vi "Default Settings.vi"(8 "error in (no error)":errorcluster, 11 "CAD Dispense2 in":refnum<class "CAD Dispense2.lvclass">) -> (0 "error out":errorcluster, 3 "CAD Dispense2 out":refnum<class "CAD Dispense2.lvclass">)   [LabVIEW 2016, in "CAD Dispense2.lvclass"]
uses:
  CAD Dispense2.lvclass
  D:/UCSB-Gantry_ms/UCSB-Gantry 0510/V5/Classes/Routine/Dispense/Dispense.lvclass
  CAD Dispense2.lvclass/CAD Dispense2.ctl
  Dispense.lvclass/Dispense.ctl
  Dispense.lvclass
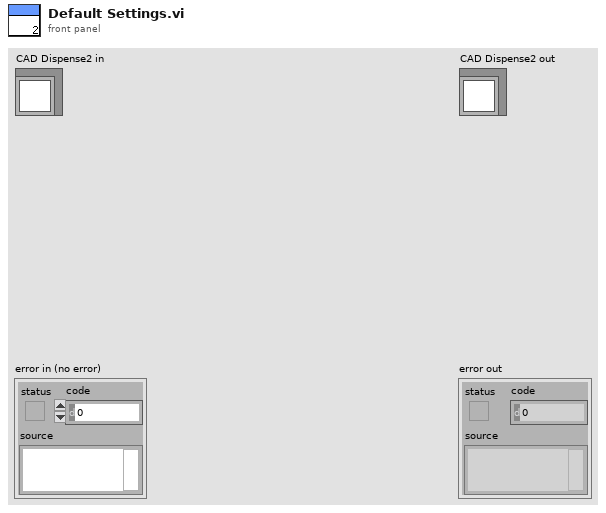
[diagram p1: front panel]
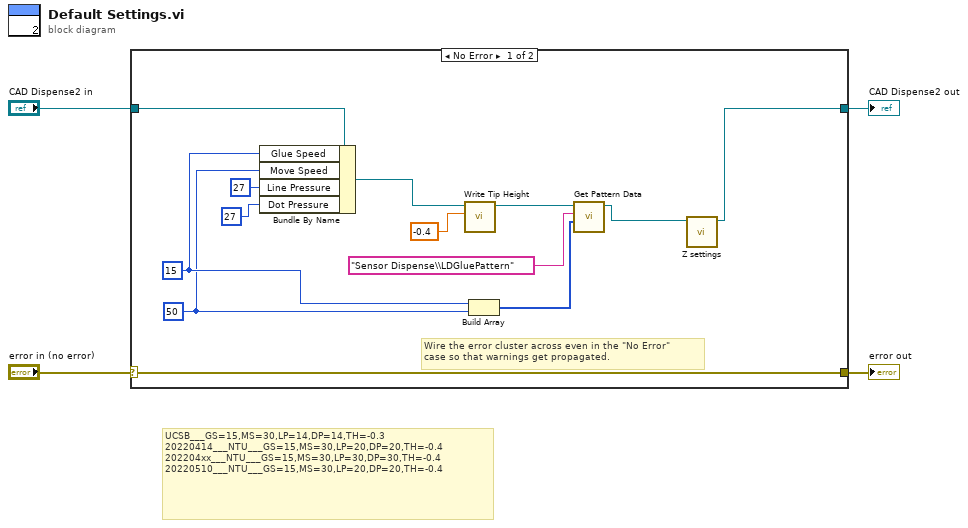
[diagram p0: block diagram]
diagram:
  # "UCSB___GS=15,MS=30,LP=14,DP=14,TH=-0.3\n20220414___NTU___GS=15,MS=30,LP=20,DP=20,TH=-0.4\n202204xx___NTU___GS=15,MS=30,LP=30,DP=30,TH=-0.4\n20220510___NTU___GS=15,MS=30,LP=20,DP=20,TH=-0.4"
  n1 = case shown="No Error" "error in (no error)" {
    selector: "error in (no error)" -> [w17 w19]
    tunnel: [w17 w19] -> w3
    tunnel: [w8 w18] -> w1
    tunnel: "CAD Dispense2 in" -> [w9 w18]
    frame No Error {
      w6 = i64 50 ("Line Pressure")
      w7 = i64 15 ("Line Pressure")
      # "Wire the error cluster across even in the \"No Error\"\ncase so that warnings get propagated."
      n2 = Bundle By Name(cluster=w9, "Glue Speed"=w7, "Move Speed"=w6, "Line Pressure"=i64 27, "Dot Pressure"=i64 27 ("Line Pressure")) -> (w13:refnum<class "CAD Dispense2.lvclass">)
      n3 = call "Write Tip Height.vi"("Tip Height"=-0.4, "Dispense in"=w13) -> ("Dispense out"=w12:refnum<class "CAD Dispense2.lvclass">)  [unwired: 8 in, 1 out]
      n4 = Build Array(w7, w6) -> (w5:i64[])
      n5 = call "Get Pattern Data.vi"("File Name"=w5, "Folder Name"="Sensor Dispense\\LDGluePattern", "Dispense.lvclass"=w12) -> ("Dispense Out"=w10:refnum<class "CAD Dispense2.lvclass">)  [unwired: 8 in]
      n6 = call-dynamic "Z settings.vi"("Dispense in"=w10) -> ("Dispense out"=w8:refnum<class "CAD Dispense2.lvclass">)  [unwired: 9 in, 1 out]
    }
    frame Error {
    }
  }
  "error out" <- w3
  "CAD Dispense2 out" <- w1
